vi "ConfigInfoTest.vi"() -> ()   [LabVIEW 2017]
uses:
  Gantry.lvclass
  Type Definitions/Virtual Modes.ctl
  FlexWorktable/FlexWorktable.lvclass
panel:
  out "homed? 2":bool
  out "homed?":bool
  out "error out":errorcluster
  in  "Config Folder":path=path "C:/Users/husker/Desktop/gantry/Config"
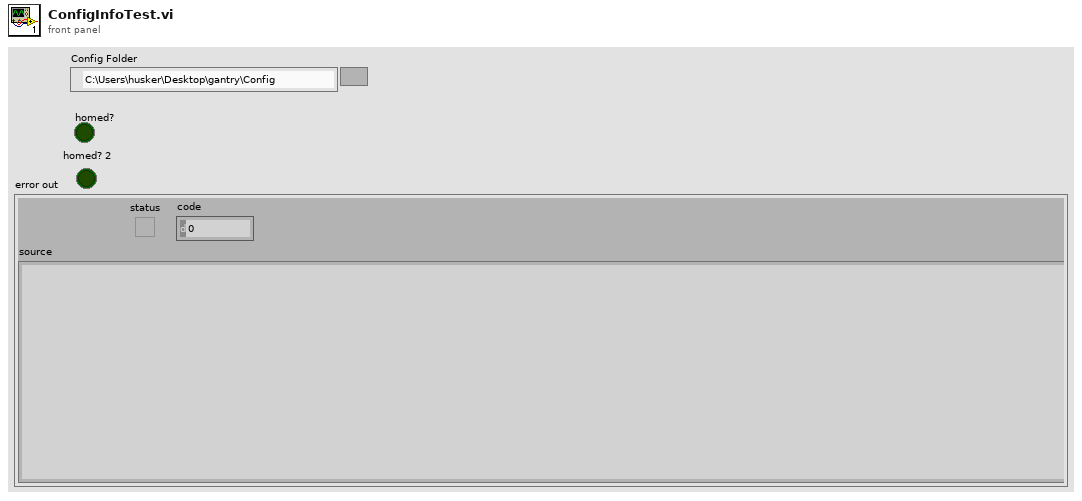
[diagram p1: front panel]
types:
  T1 = typedef "Virtual Modes.ctl" = enum16{"Nonvirtual", "Virtual"}
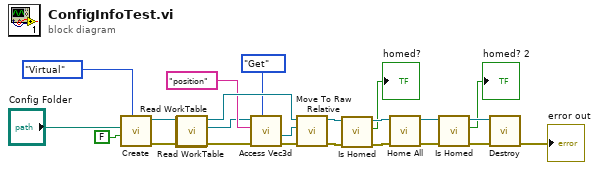
[diagram p0: block diagram]
diagram:
  n1 = call "Create.vi"("Virtual Mode"=Virtual_Modes."Virtual", "HOME?"=FALSE, "Config Folder"="Config Folder") -> ("error out"=w10:errorcluster, "Gantry out"=w9:refnum<class "Gantry.lvclass">)  [unwired: 6 in, 1 out]
  n2 = call-dynamic "Read WorkTable.vi"() -> ()  [unwired: 9 in, 3 out]
  n3 = call-dynamic "Read WorkTable.vi"("error in"=w10, "Gantry Class in"=w9) -> ("error out"=w6:errorcluster, "Worktable"=w4:refnum<class "FlexWorktable.lvclass">, "Gantry Class out"=w11:refnum<class "Gantry.lvclass">)  [unwired: 7 in]
  n4 = call-dynamic "Access Vec3d.vi"("Get/Set"=enum16{"Get", "Set"}."Get", "error in (no error)"=w6, "Key"="position", "FlexWorktable in"=w4) -> ("error out"=w3:errorcluster, "Value out"=w2:refnum<class "Vec3d.lvclass">)  [unwired: 5 in, 1 out]
  n5 = call-dynamic "Move To Raw Relative.vi"("error in"=w3, "Delta"=w2, "Gantry in"=w11) -> ("error out"=w14:errorcluster, "Gantry out"=w15:refnum<class "Gantry.lvclass">)  [unwired: 7 in]
  n6 = call "Is Homed.vi"("error in (no error)"=w14, "Gantry in"=w15) -> ("error out"=w12:errorcluster, "homed?"=→"homed?":bool, "Gantry out"=w17:refnum<class "Gantry.lvclass">)  [unwired: 7 in]
  n7 = call "Home All.vi"("error in (no error)"=w12, "Gantry in"=w17) -> ("error out"=w19:errorcluster, "Gantry out"=w21:refnum<class "Gantry.lvclass">)  [unwired: 8 in]
  n8 = call "Is Homed.vi"("error in (no error)"=w19, "Gantry in"=w21) -> ("error out"=w18:errorcluster, "homed?"=→"homed? 2":bool, "Gantry out"=w20:refnum<class "Gantry.lvclass">)  [unwired: 7 in]
  n9 = call "Destroy.vi"("error in"=w18, "Gantry Class in"=w20) -> ("error out"=→"error out":errorcluster)  [unwired: 9 in]
